vi "EndingGame.vi"(7 "VI Refnum":refnum<vi>, 8 "Error In":errorcluster, 10 "EndData":T1, 11 "MainData":T3) -> (0 "Error Out":errorcluster, 2 "PlayAgain":bool)   [LabVIEW 2020]
doc: "Dialog with game result."
uses:
  typeDef/MainDataCluster.ctl
  <vilib>/picture/picture.llb/imagedata.ctl
  typeDef/StateMachineEnum.ctl
  typeDef/EventData.ctl
  typeDef/EndType.ctl
panel:
  out "ResultInfo":string
  in  "Play":bool
  in  "Stop":bool
  # "Chcesz spróbowaæ jeszcze raz ?"
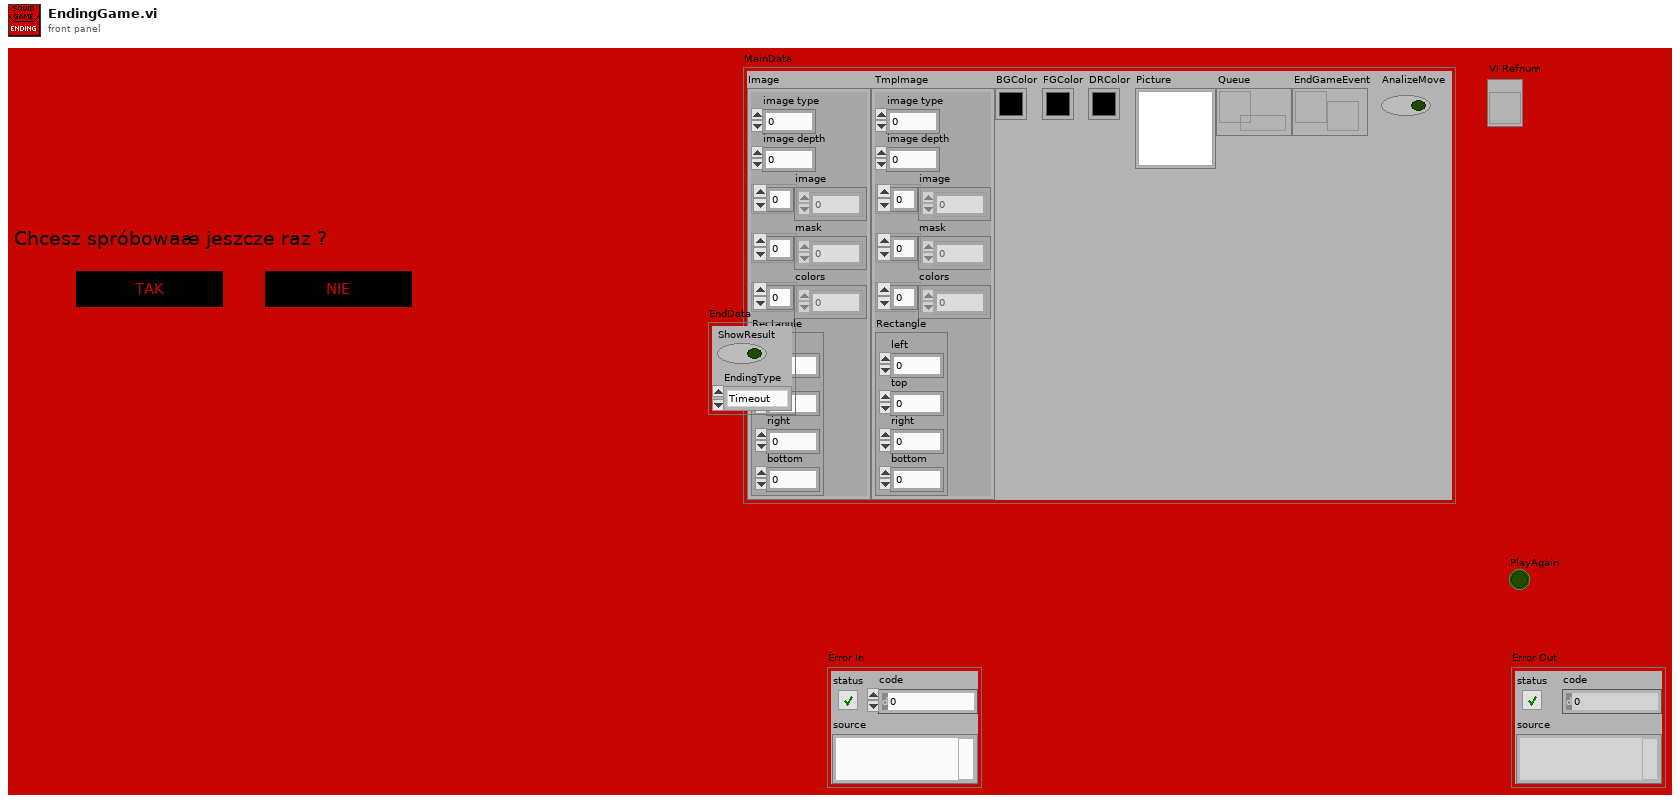
[diagram p1: front panel]
types:
  T1 = typedef "EventData.ctl" = cluster{"ShowResult":bool, "EndingType":T2}
  T2 = typedef "EndType.ctl" = enum16{"Timeout", "MouseUp", "OutOfLine", "CloseLine", "UserEnd"}
  T3 = typedef "MainDataCluster.ctl" = cluster{"Image":T4, " TmpImage":T4, "BGColor":u32, "FGColor":u32, "DRColor":u32, "Picture":picture, "Queue ":refnum<queue>, "EndGameEvent":refnum<user-event>, "AnalizeMove":bool}
  T4 = typedef "imagedata.ctl" = cluster{"image type":i32, "image depth":i32, "image":u8[], "mask":u8[], "colors":u32[], "Rectangle":cluster{"left":i16, "top":i16, "right":i16, "bottom":i16}}
  T5 = enum32{"Invalid", "Standard", "Closed", "Hidden", "Minimized", "Maximized"}
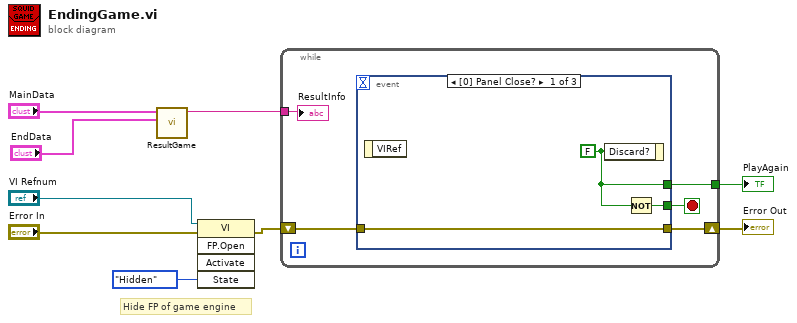
[diagram p0: block diagram]
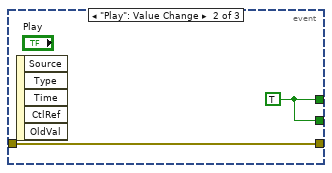
[diagram p2: hidden frame]
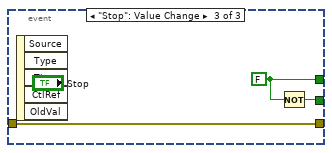
[diagram p3: hidden frame]
diagram:
  # "Hide FP of game engine"
  n1 = call "ResultGame.vi"("EndData"="EndData", "MainData"="MainData") -> ("Result info"=w3:string)  [unwired: 9 in]
  n2 = invoke class="VI" method="FP.Open"(reference="VI Refnum", error in="Error In", "State"=T5."Hidden") -> (error out=w6:errorcluster)  [unwired: 2 in, 4 out]
  n3 = while {
    shift-right: [w12] -> w5
    shift-left: w6 -> [w13]
    tunnel: [w14] -> w4
    tunnel: w3 -> [w10]
    stop <- w11 stop-if-true
    n4 = event shown="[0] Panel Close?" {
      selector: _ -> [_ _ _]
      dyn-events: _ -> [_ _ _]
      timeout: _ -> [_ _ _]
      tunnel: [w16 w18 w21] -> w14
      tunnel: w13 -> [w17 w19 w22]
      tunnel: [w17 w19 w22] -> w12
      tunnel: [w15 w18 w20] -> w11
      event Panel Close? {
        w16 = FALSE ("Discard?")
        n5 = event-data() -> ()  [unwired: 1 in, 1 out]
        n6 = event-data("Discard?"=w16) -> ()  [unwired: 1 in, 1 out]
        n7 = Not(x=w16) -> (.not. x?=w15:bool)
      }
      event "Play": Value Change {
        w18 = TRUE
        n8 = event-data() -> ()  [unwired: 1 in, 5 out]
      }
      event "Stop": Value Change {
        w21 = FALSE
        n9 = event-data() -> ()  [unwired: 1 in, 5 out]
        n10 = Not(x=w21) -> (.not. x?=w20:bool)
      }
    }
    "ResultInfo" <- w10
  }
  "PlayAgain" <- w4
  "Error Out" <- w5
